vi "Dashboard Main.vi"() -> ()   [LabVIEW 2011]
uses:
  <vilib>/Rock Robotics/WPI/DriverStation/WPI_DriverStationDigitalData.ctl
panel:
  out "Processed Image":T1(plugin-control)
  out "8 -- Battery":sgl(graph)
  out "Analog Input":sgl[](array[slide]) scale=0.0..5.0
  in  "Viewer":enum32{"Camera Image", "Kinect Skeleton"}(tab)
  in  "Video Enable":bool=TRUE
  out "Camera Image":T1(plugin-control)
  out "Buttons 1":cluster{"1":bool, "2":bool, "3":bool}
  out "Kinect 1":cluster{"X":dbl, "Y":dbl, "Z":dbl} {"X" scale=1.0..-1.0; "Y" scale=1.0..-1.0; "Z" scale=1.0..-1.0}
  out "Buttons 2":cluster{"1":bool, "2":bool, "3":bool}
  out "Kinect 2":cluster{"X":dbl, "Y":dbl, "Z":dbl} {"X" scale=1.0..-1.0; "Y" scale=1.0..-1.0; "Z" scale=1.0..-1.0}
  out "Version":string
  out "Skeleton Picture":picture
  out "Players":i8
  out "Dashboard Datatype Warning":string="Warning: The Dashboard Datatype used by the robot project and this dashboard do not match.\nSee diagram for more details."
  out "Robot IP Address":string
  out "Image Error Message":string="Timeout in Camera Communications"
  out "Solenoid Output":bool[](array[boolean])
  out "PWM":cluster{u8, u8}[](array[slide])=[{0, 157}, {0, 157}, {0, 157}, {0, 157}, {0, 157}, {0, 157}, {0, 157}, {0, 157}, {0, 157}, {0, 169}] scale=1.0..255.0
  out "GPIO Output Enable":bool[](array[boolean])
  out "GPIO State":bool[](array[boolean])
  out "Relay":cluster{"Forward":bool[], "Reverse":bool[]}
  # "Analog #1"
  # "1"
  # "7"
  # "Communications"
  # "Solenoid #1"
  # "1"
  # "8"
  # "Digital #1"
  # "1"
  # "10"
  # "1"
  # "14"
  # "1"
  # "8"
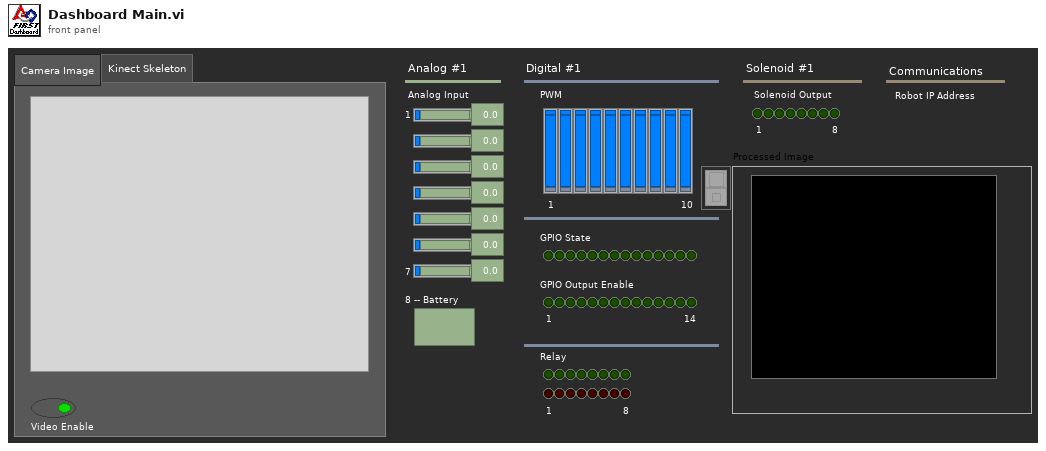
[diagram p1: front panel]
types:
  T1 = typedef "IMAQ Image.ctl" = refnum<image>
  T2 = typedef "WPI_DriverStationDigitalData.ctl" = cluster{"Relay Fwd":u8, "Relay Rev":u8, "GPIO":u16, "GPIO_OE":u16, "PWM":cluster{"PWM[0]":u8, "PWM[1]":u8, "PWM[2]":u8, "PWM[3]":u8, "PWM[4]":u8, "PWM[5]":u8, "PWM[6]":u8, "PWM[7]":u8, "PWM[8]":u8, "PWM[9]":u8}}
  T3 = cluster{cluster{"AnalogModule[0]":cluster{"Channel[0]":sgl, "Channel[1]":sgl, "Channel[2]":sgl, "Channel[3]":sgl, "Channel[4]":sgl, "Channel[5]":sgl, "Channel[6]":sgl, "Channel[7]":sgl}, "AnalogModule[1]":cluster{"Channel[0]":sgl, "Channel[1]":sgl, "Channel[2]":sgl, "Channel[3]":sgl, "Channel[4]":sgl, "Channel[5]":sgl, "Channel[6]":sgl, "Channel[7]":sgl}}, cluster{"DigitalModule[0]":T2, "DigitalModule[1]":T2}, "Solenoid":u8}
  T4 = typedef "Image Type" = u32
  T5 = cluster{"Competition mode":bool, "Robot Link":bool, "Autonomous":bool, "Enabled":bool, "E-Stop":bool}
  T6 = cluster{"AnalogModule[0]":cluster{"Channel[0]":sgl, "Channel[1]":sgl, "Channel[2]":sgl, "Channel[3]":sgl, "Channel[4]":sgl, "Channel[5]":sgl, "Channel[6]":sgl, "Channel[7]":sgl}, "AnalogModule[1]":cluster{"Channel[0]":sgl, "Channel[1]":sgl, "Channel[2]":sgl, "Channel[3]":sgl, "Channel[4]":sgl, "Channel[5]":sgl, "Channel[6]":sgl, "Channel[7]":sgl}}
  T7 = cluster{"DigitalModule[0]":T2, "DigitalModule[1]":T2}
  T8 = cluster{"Channel[0]":sgl, "Channel[1]":sgl, "Channel[2]":sgl, "Channel[3]":sgl, "Channel[4]":sgl, "Channel[5]":sgl, "Channel[6]":sgl, "Channel[7]":sgl}[]
  T9 = cluster{"Channel[0]":sgl, "Channel[1]":sgl, "Channel[2]":sgl, "Channel[3]":sgl, "Channel[4]":sgl, "Channel[5]":sgl, "Channel[6]":sgl, "Channel[7]":sgl}
  T10 = typedef "LVRectTypeDef.ctl" = cluster{"left":i16, "top":i16, "right":i16, "bottom":i16}
  T11 = typedef "SkeletonTrackState.ctl" = enum32{"NotTracked", "PositionOnly", "Tracked"}
  T12 = cluster{"TrackingState":u8[], "Position":cluster{"x":sgl, "y":sgl, "z":sgl}, cluster{"x":sgl, "y":sgl, "z":sgl, sgl}[], "TrackState":T11}
  T13 = cluster{cluster{"ScaledToPercentRange":dbl, "ScaledToPercentRange":dbl, "ScaledToPercentRange":dbl}, cluster{bool, bool, bool}}[]
  T14 = typedef "LVBoundsTypeDef.ctl" = cluster{"Width":u32, "Height":u32}
  T15 = cluster{cluster{"ScaledToPercentRange":dbl, "ScaledToPercentRange":dbl, "ScaledToPercentRange":dbl}, cluster{bool, bool, bool}}
  T16 = cluster{"ScaledToPercentRange":dbl, "ScaledToPercentRange":dbl, "ScaledToPercentRange":dbl}
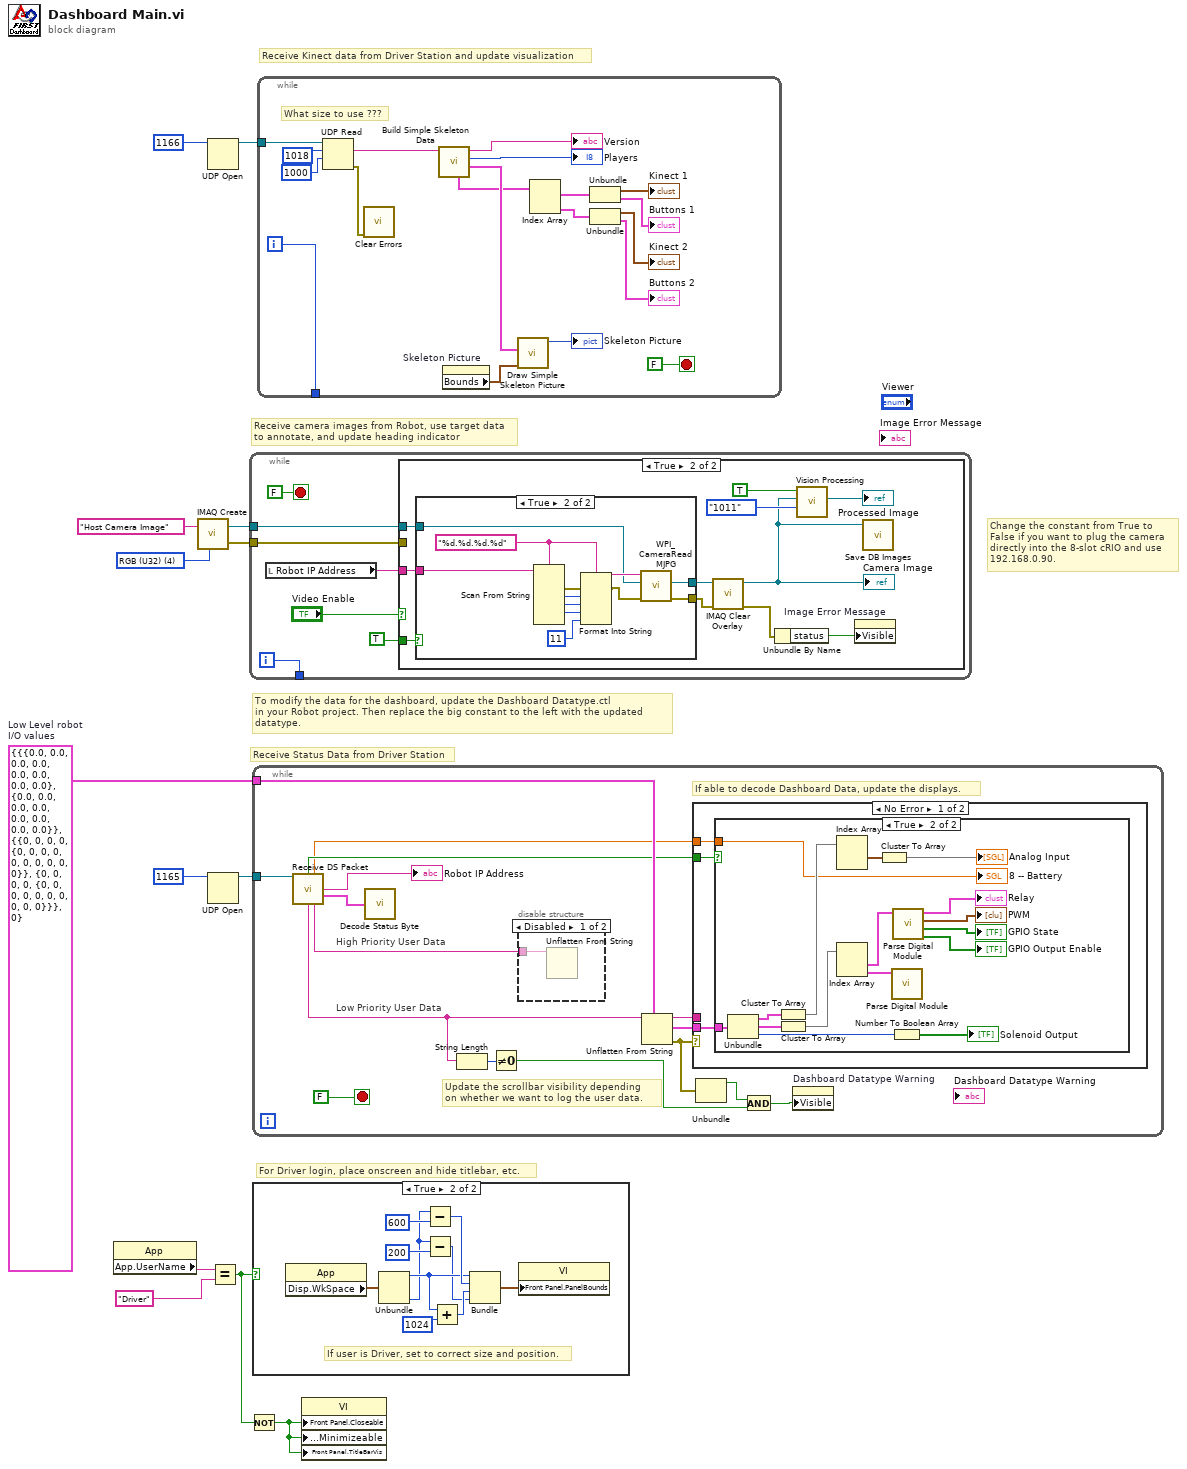
[diagram p0: block diagram]
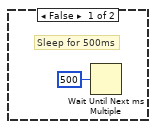
[diagram p6: hidden frame]
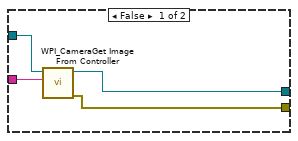
[diagram p7: hidden frame]
diagram:
  w3 = T3 {{"AnalogModule[0]"={"Channel[0]"=0.0, "Channel[1]"=0.0, "Channel[2]"=0.0, "Channel[3]"=0.0, "Channel[4]"=0.0, "Channel[5]"=0.0, "Channel[6]"=0.0, "Channel[7]"=0.0}, "AnalogModule[1]"={"Channel[0]"=0.0, "Channel[1]"=0.0, "Channel[2]"=0.0, "Channel[3]"=0.0, "Channel[4]"=0.0, "Channel[5]"=0.0, "Channel[6]"=0.0, "Channel[7]"=0.0}}, {"DigitalModule[0]"={"Relay Fwd"=0, "Relay Rev"=0, "GPIO"=0, "GPIO_OE"=0, "PWM"={"PWM[0]"=0, "PWM[1]"=0, "PWM[2]"=0, "PWM[3]"=0, "PWM[4]"=0, "PWM[5]"=0, "PWM[6]"=0, "PWM[7]"=0, "PWM[8]"=0, "PWM[9]"=0}}, "DigitalModule[1]"={"Relay Fwd"=0, "Relay Rev"=0, "GPIO"=0, "GPIO_OE"=0, "PWM"={"PWM[0]"=0, "PWM[1]"=0, "PWM[2]"=0, "PWM[3]"=0, "PWM[4]"=0, "PWM[5]"=0, "PWM[6]"=0, "PWM[7]"=0, "PWM[8]"=0, "PWM[9]"=0}}}, "Solenoid"=0}  # Low Level robot I/O values
  w11 = T4 4 items=["Grayscale (U8)", "Grayscale (I16)", "Grayscale (SGL)", "Complex (CSG)", "RGB (U32)", "HSL (U32)", "RGB (U64)"] ("Image Type")
  # "Change the constant from True to\nFalse if you want to plug the camera\ndirectly into the 8-slot cRIO and use\n192.168.0.90."
  # "Receive Kinect data from Driver Station and update visualization"
  # "For Driver login, place onscreen and hide titlebar, etc."
  # "To modify the data for the dashboard, update the Dashboard Datatype.ctl\nin your Robot project. Then replace the big constant to the left with the updated\ndatatype."
  # "Receive Status Data from Driver Station"
  # "Receive camera images from Robot, use target data\nto annotate, and update heading indicator"
  n1 = property class="App"() -> ("App.UserName"=w6:string)  [unwired: 2 in, 2 out]
  n2 = call "IMAQ Create"("Image Name"="Host Camera Image", "Image Type"=w11) -> ("New Image"=w9:T1, "error out"=w8:errorcluster)  [unwired: 2 in, 1 out]
  n3 = UDP Open(11:u16 1166 ("port")) -> (port=w1:refnum<k16>)  [unwired: 2 in, 4 out]
  n4 = UDP Open(11:u16 1165 ("port")) -> (port=w12:refnum<k16>)  [unwired: 2 in, 4 out]
  n5 = Equal?(x=w6, y="Driver") -> (x = y?=w5:bool)
  n6 = Not(x=w5) -> (.not. x?=w4:bool)
  n7 = while {
    tunnel: w9 -> [w18]
    tunnel: w8 -> [w14]
    tunnel: [w15] -> _
    i -> [w15]
    stop <- FALSE stop-if-true
    n8 = local read "Robot IP Address"() -> (w19:string)
    n9 = case shown="True" "Video Enable" {
      tunnel: w19 -> [_ w32]
      tunnel: w18 -> [_ w31]
      tunnel: TRUE -> [_ w28]
      tunnel: w14 -> [_ _]
      frame False {
        # "Sleep for 500ms"
        n10 = Wait Until Next ms Multiple(millisecond multiple=u32 500) -> ()  [unwired: 1 out]
      }
      frame True {
        n11 = case shown="True" w28 {
          tunnel: w31 -> [w35 w42]
          tunnel: [w33 w40] -> w23
          tunnel: [w34 w41] -> w29
          tunnel: w32 -> [w36 w45]
          frame False {
            n12 = call <vilib>:"WPI_CameraGet Image From Controller.vi"("Controller Address"=w36, "Image"=w35) -> ("error out"=w33:errorcluster, "Image Out"=w34:T1)  [unwired: 2 in, 6 out]
          }
          frame True {
            w37 = "%d.%d.%d.%d" ("format string")
            n13 = Scan From String(format string=w37, input string=w45) -> (error out=w44:errorcluster, output 1=w46:i32, output 2=w47:i32, output 3=w48:i32)  [unwired: 2 in, 7 out]
            n14 = Format Into String(format string=w37, error in=w44, w46, w47, w48, 11 ("IP Suffix:")) -> (resulting string=w43:string, error out=w39:errorcluster)  [unwired: 1 in]
            n15 = call <vilib>:"WPI_CameraRead MJPG.vi"("error in"=w39, "Image"=w42, "address"=w43) -> ("error out"=w40:errorcluster, "Image Out"=w41:T1)  [unwired: 7 in]
          }
        }
        n16 = call "IMAQ Clear Overlay"("error in (no error)"=w23, "Image"=w29) -> ("error out"=w27:errorcluster, "Image Out"=w24:T1)  [unwired: 1 in, 7 out]
        "Camera Image" <- w24
        n17 = Unbundle By Name(w27) -> ("status"=w30:bool)
        n18 = call "Vision Processing.vi"("Camera Type"=enum16{"206", "1011"}."1011", "Input Image"=w24, "Enable Vision"=TRUE) -> ("Processed Image"=→"Processed Image":T1)  [unwired: 4 in]
        n19 = property on="Image Error Message" class="Str"("Visible"=w30) -> ()  [unwired: 2 in, 2 out]
        n20 = call "Save DB Images.vi"("Image"=w24) -> ()  [unwired: 2 in, 1 out]
      }
    }
  }
  n21 = while {
    tunnel: w12 -> [w62]
    tunnel: w3 -> [w61]
    stop <- FALSE stop-if-true
    # "High Priority User Data"
    # "Low Priority User Data"
    # "Update the scrollbar visibility depending\non whether we want to log the user data."
    # "If able to decode Dashboard Data, update the displays."
    n22 = call "Receive DS Packet.vi"("Recv Socket"=w62) -> ("New Dashboard Data"=w58:bool, "Battery"=w49:sgl, "Robot IP Address"=→"Robot IP Address":string, "Status"=w63:T5, "Low Priority User Data"=w51:string, "High Priority User Data"=w50:string)  [unwired: 1 in, 8 out]
    n23 = call "Decode Status Byte.vi"("Status Byte"=w63) -> ()  [unwired: 2 out]
    n24 = String Length(string=w51) -> (length=w53:i32)
    n25 = Not Equal To 0?(x=w53) -> (x != 0?=w56:bool)
    n26 = disable-structure shown="Disabled" {
      disable-tunnel: w50 -> [w65 _]
      frame Disabled {
        n27 = Unflatten From String(binary string=w65) -> ()  [unwired: 2 in, 5 out]
      }
      frame Enabled {
      }
    }
    n28 = Unflatten From String(type=w61, binary string=w51) -> (rest of the binary string=w54:string, value=w60:T3, error out=w59:errorcluster)  [unwired: 1 in, 2 out]
    n29 = case shown="No Error" w59 {
      tunnel: w60 -> [w68 _]
      tunnel: w58 -> [w67 _]
      tunnel: w54 -> [_ _]
      tunnel: w49 -> [w66 _]
      frame No Error {
        n30 = case shown="True" w67 {
          tunnel: w68 -> [_ w75]
          tunnel: w66 -> [_ w69]
          frame False {
            # "Don't update if the robot hasn't sent new data"
          }
          frame True {
            n31 = Unbundle(w75) -> (w72:T6, w73:T7, "Solenoid"=w74:u8)
            n32 = Cluster To Array(cluster=w72) -> (array=w83:T8)
            n33 = Cluster To Array(cluster=w73) -> (array=w82:T2[])
            n34 = Index Array(array=w83) -> (element #1=w70:T9)  [unwired: 2 in, 1 out]
            n35 = Index Array(array=w82) -> (element #1=w81:T2, element #2=w76:T2)  [unwired: 2 in]
            n36 = Cluster To Array(cluster=w70) -> (array=→"Analog Input":sgl[])
            n37 = call "Parse Digital Module.vi"("DigitalModule"=w76) -> ()  [unwired: 11 out]
            n38 = Number To Boolean Array(number=w74) -> (Boolean array=→"Solenoid Output":bool[])
            n39 = call "Parse Digital Module.vi"("DigitalModule"=w81) -> ("GPIO Output Enable"=→"GPIO Output Enable":bool[], "GPIO State"=→"GPIO State":bool[], "PWM"=→"PWM":cluster{u8, u8}[], "Relay"=→"Relay":cluster{"Forward":bool[], "Reverse":bool[]})  [unwired: 7 out]
            "8 -- Battery" <- w69
          }
        }
      }
      frame Error {
        # "Your datatypes don't match. The Dashboard Datatype.ctl in your Robot project\nand the big constant to the left of the loop need to match."
      }
    }
    n40 = Unbundle(w59) -> ("status"=w55:bool)  [unwired: 2 out]
    n41 = And(x=w55, y=w56) -> (x .and. y?=w57:bool)
    n42 = property on="Dashboard Datatype Warning" class="Str"("Visible"=w57) -> ()  [unwired: 2 in, 2 out]
  }
  n43 = case shown="True" w5 {
    frame False {
    }
    frame True {
      # "If user is Driver, set to correct size and position."
      n44 = property class="App"() -> ("Disp.WkSpace"=w94:T10)  [unwired: 2 in, 2 out]
      n45 = Unbundle(w94) -> ("left"=w89:i16, "bottom"=w85:i16)  [unwired: 2 out]
      n46 = Subtract(x=w85, y=600) -> (x-y=w91:i32)
      n47 = Subtract(x=w85, y=200) -> (x-y=w86:i32)
      n48 = Add(x=w89, y=1024) -> (x+y=w90:i32)
      n49 = Bundle("left"=w89, w91, w90, w86) -> (w93:cluster{"left":i16, i32, i32, i32})  [unwired: 1 out]
      n50 = property class="VI"("Front Panel.PanelBounds"=w93) -> ()  [unwired: 2 in, 2 out]
    }
  }
  n51 = while {
    tunnel: w1 -> [w111]
    tunnel: [w95] -> _
    i -> [w95]
    stop <- FALSE stop-if-true
    # "What size to use ???"
    n52 = UDP Read(connection ID=w111, max size (548)=1018 ("bytes to read"), timeout ms (25000)=1000) -> (data out=w105:string, error out=w103:errorcluster)  [unwired: 1 in, 3 out]
    n53 = call <vilib>:"Clear Errors.vi"("error in (no error)"=w103) -> ()  [unwired: 6 in, 1 out]
    n54 = call "Build Simple Skeleton Data.vi"("data out"=w105) -> ("Skeleton Data"=w106:T12, "NumPlayers"=→"Players":i8, "Version String"=→"Version":string, "Simple Joystick Info"=w102:T13)  [unwired: 6 in, 1 out]
    n55 = property on="Skeleton Picture" class="Pict"() -> ("Bounds"=w107:T14)  [unwired: 2 in, 2 out]
    n56 = call "Draw Simple Skeleton Picture.vi"("Bounds"=w107, "Simple Skeleton"=w106) -> ("new picture out"=→"Skeleton Picture":picture)  [unwired: 9 in]
    n57 = Index Array(array=w102) -> (element #1=w101:T15, element #2=w100:T15)  [unwired: 2 in]
    n58 = Unbundle(w101) -> (→"Kinect 1":T16, →"Buttons 1":cluster{bool, bool, bool})
    n59 = Unbundle(w100) -> (→"Kinect 2":T16, →"Buttons 2":cluster{bool, bool, bool})
  }
  n60 = property class="VI"("Front Panel.Closeable"=w4, "Front Panel.Minimizeable"=w4, "Front Panel.TitleBarVis"=w4) -> ()  [unwired: 2 in, 2 out]
